vi "Launch Module.vi"(8 "error in":errorcluster, 10 "Target UDP connection ref":refnum<k16>, 11 "IP:Port:Master/Slave":string) -> (0 "error out":errorcluster, 3 "IP:Port:Master/Slave out":string)   [LabVIEW 2021, in "RT Interpreter.lvlib"]
uses:
  RT Interpreter.lvlib
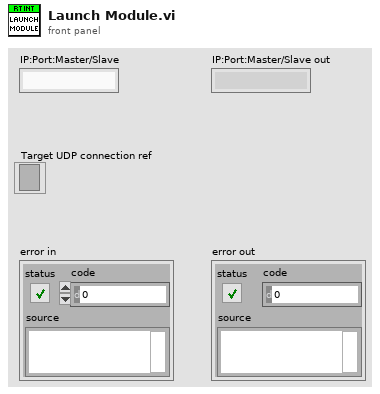
[diagram p1: front panel]
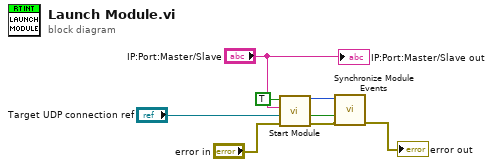
[diagram p0: block diagram]
diagram:
  n1 = call "Start Module.vi"("error in"="error in", "Target UDP connection ref"="Target UDP connection ref", "IP:Port:Master/Slave"="IP:Port:Master/Slave", "Run as Singleton? (F)"=TRUE) -> ("error out"=w8:errorcluster, "Wait for Event Sync?"=w6:bool, "Module ID"=w7:i32)  [unwired: 3 in, 2 out]
  n2 = call "Synchronize Module Events.vi"("error in"=w8, "Wait for Event Sync?"=w6, "Module ID in"=w7) -> ("error out"=→"error out":errorcluster)  [unwired: 7 in, 1 out]
  "IP:Port:Master/Slave out" <- "IP:Port:Master/Slave"
